vi "Errorbar2010.vi"   [LabVIEW 2013]
uses:
  <vilib>/Heliosphere Research LLC/Advanced Plotting Toolkit/api_plotting/ErrorbarProperties.ctl
  <vilib>/Heliosphere Research LLC/Advanced Plotting Toolkit/typedefs/PlotColor.ctl
  <vilib>/Heliosphere Research LLC/Advanced Plotting Toolkit/properties/Display.ctl
  ModeType.ctl
  <vilib>/Heliosphere Research LLC/Advanced Plotting Toolkit/Advanced Plotting Toolkit.lvlib
types:
  T1 = typedef "ModeType.ctl" = enum16{"Normal", "Expected Failure", "Skipped", "Broken"}
  T2 = typedef "Advanced Plotting Toolkit.lvlib/ErrorbarProperties.ctl" = cluster{"Color":T3, "Line Width":dbl, "Cap Size":dbl, "Display":T4}
  T3 = typedef "Advanced Plotting Toolkit.lvlib/PlotColor.ctl" = u32
  T4 = typedef "Advanced Plotting Toolkit.lvlib/Display.ctl" = cluster{"Alpha":dbl, "Z Order":dbl}
  T5 = typedef "Advanced Plotting Toolkit.lvlib/PlotID.ctl" = i32
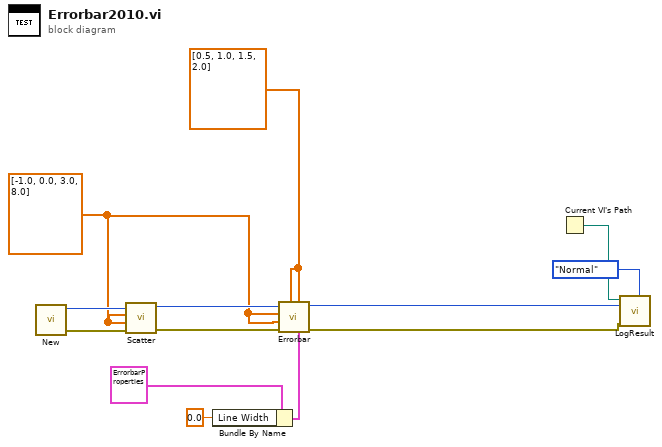
[diagram p0: block diagram]
diagram:
  w5 = dbl[] [0.5, 1.0, 1.5, 2.0] ("X Errors")
  w6 = dbl[] [-1.0, 0.0, 3.0, 8.0] ("X Data")
  n1 = call <vilib>:"New.vi"() -> ("error out"=w7:errorcluster, "Plot ID"=w10:T5)  [unwired: 10 in]
  n2 = call <vilib>:"Scatter.vi"("error in (no error)"=w7, "Y Data"=w6, "X Data"=w6, "Plot ID"=w10) -> ("error out"=w8:errorcluster, "Plot ID Out"=w9:T5)  [unwired: 6 in]
  n3 = Bundle By Name(cluster=T2 {"Color"=2147483647, "Line Width"=nan, "Cap Size"=nan, "Display"={"Alpha"=nan, "Z Order"=nan}} ("Errorbar Properties"), "Line Width"=0.0) -> (w3:T2)
  n4 = call <vilib>:"Errorbar.vi"("Properties"=w3, "Y Errors"=w5, "X Errors"=w5, "error in (no error)"=w8, "Y Data"=w6, "X Data"=w6, "Plot ID"=w9) -> ("error out"=w11:errorcluster, "Plot ID out"=w12:T5)  [unwired: 3 in]
  n5 = Current VI's Path() -> (path=w13:path)
  n6 = call "LogResult.vi"("Mode"=ModeType."Normal", "Test Result"=w11, "Test Artifact"=w12, "VI Path"=w13) -> ()  [unwired: 8 in]
